vi "path_output.vi"() -> (0 "Path output":path caption="selected path")   [LabVIEW 2016]
doc: "This vi inisilizes the path output and the text name then returns the path output.\n\nMuhannad Alghamdi\nCSUSB Physics 350"
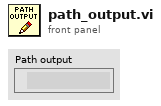
[diagram p1: front panel]
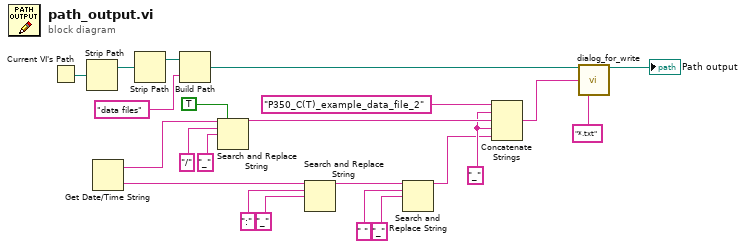
[diagram p0: block diagram]
diagram:
  w8 = "_" ("string")
  n1 = Current VI's Path() -> (path=w6:path)
  n2 = Strip Path(path=w6) -> (stripped path=w1:path)  [unwired: 1 out]
  n3 = Get Date/Time String() -> (date string=w19:string, time string=w15:string)  [unwired: 3 in]
  n4 = Strip Path(path=w1) -> (stripped path=w2:path)  [unwired: 1 out]
  n5 = Build Path(base path=w2, name or relative path="data files") -> (appended path=w4:path)
  n6 = Search and Replace String(replace all?=TRUE ("replace all? (F)"), input string=w19, search string="/", replace string="_" ("replace string (\"\")")) -> (result string=w17:string)  [unwired: 4 in, 3 out]
  n7 = Search and Replace String(input string=w15, search string=":", replace string="_" ("replace string (\"\")")) -> (result string=w9:string)  [unwired: 5 in, 3 out]
  n8 = Search and Replace String(input string=w9, search string=" ", replace string="_" ("replace string (\"\")")) -> (result string=w7:string)  [unwired: 5 in, 3 out]
  n9 = Concatenate Strings("P350_C(T)_example_data_file_2" ("string"), w8, w17, w8, w7) -> (w20:string)
  n10 = call "dialog_for_write.vi"("start path"=w4, "default name"=w20, "pattern (all files)"="*.txt") -> ("selected path"=→"Path output":path)  [unwired: 9 in, 3 out]
